vi "03_Perioda_frekvence_ze_spektra.vi"() -> ()   [LabVIEW 2019]
uses:
  <vilib>/Analysis/2dsp.llb/Real FFT.vi
  <vilib>/measure/NI_MABase.lvlib
  <vilib>/Analysis/NI_AALPro.lvlib
panel:
  out "Perioda signalu (s)":dbl=0.041666666666666664
  out "Frekvence signalu (Hz)":dbl=24.0
  out "SS (V)":dbl=2.573496971081113e-16
  in  "offset":dbl format="%0.2p"
  out "Spektrum":cluster{dbl[], dbl[]}(graph)
  out "Rozliseni a presnost spektra (Hz)":dbl=1.0
  out "Casovy prubeh":cluster{dbl[], dbl[]}(graph)
  out "dt (s)":dbl=0.0005
  out "Vzorkovaci Frekvence (N)":dbl=2000.0
  in  "Amplituda sumu":dbl format="%.2p"
  in  "Info o vzorkovani":T1={"Vzorkovaci frekvence"=2000.0, "Pocet vzorku v okne"=2000.0} {"Vzorkovaci frekvence" format="%.2p"}
  in  "Faze":dbl format="%.2p"
  in  "Amplituda":dbl=10.0 format="%0.2p"
  in  "Frekvence":dbl=24.0 format="%0.2p"
  # "GENEROVANI SIGNALU"
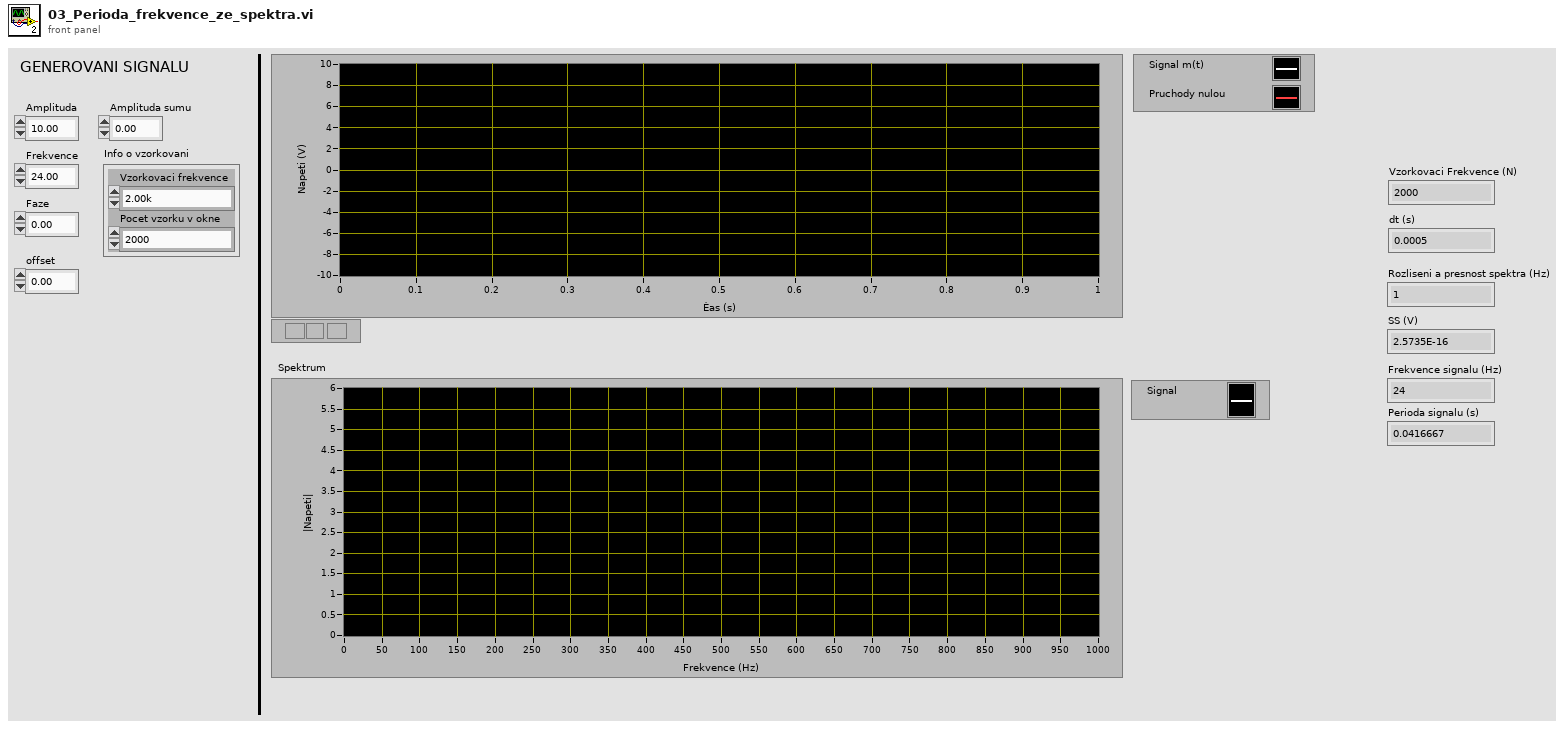
[diagram p1: front panel]
types:
  T1 = cluster{"Vzorkovaci frekvence":dbl, "Pocet vzorku v okne":dbl}
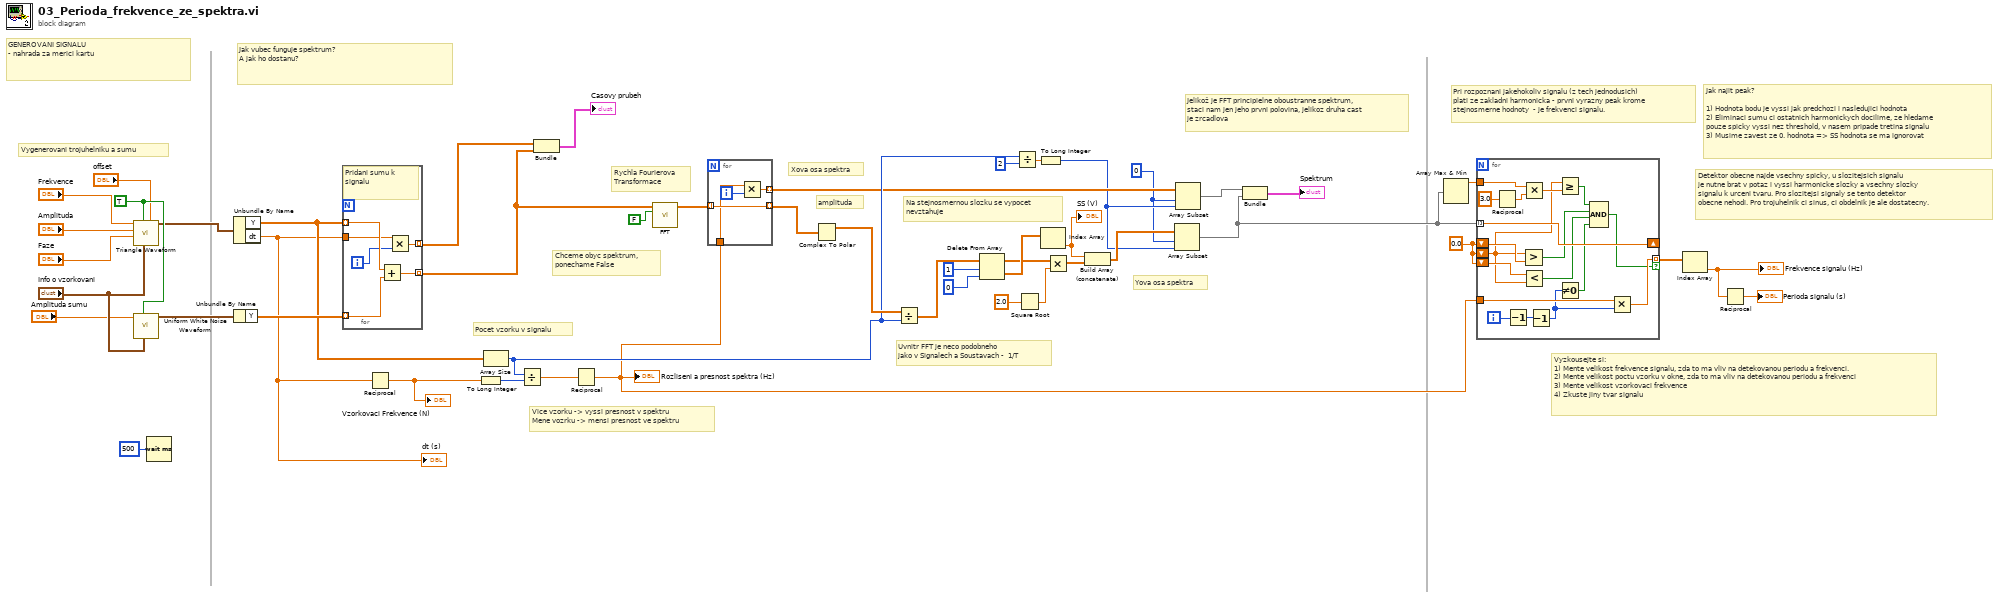
[diagram p0: block diagram]
diagram:
  w7 = 0.0
  w8 = 0 ("index")
  w43 = TRUE ("reset signal")
  # "Vyzkousejte si:\n1) Mente velikost frekvence signalu, zda to ma vliv na detekovanou periodu a frekvenci.\n2) Mente velikost poctu vzorku v okne, zda to ma vliv na detekovanou periodu a frekvenci\n3) Mente velikost vzorkovaci frekvence\n4) Zkuste jiny tvar signalu"
  # "Detektor obecne najde vsechny spicky, u slozitejsich signalu\nje nutne brat v potaz i vyssi harmonicke slozky a vsechny slozky\nsignalu k urceni tvaru. Pro slozitejsi signaly se tento detektor\nobecne nehodi. Pro trojuhelnik ci sinus, ci obdelnik je ale dostatecny."
  # "Jak najit peak?\n\n1) Hodnota bodu je vyssi jak predchozi i nasledujici hodnota\n2) Eliminaci sumu ci ostatnich harmonickych docilime, ze hledame\npouze spicky vyssi nez threshold, v nasem pripade tretina signalu\n3) Musime zavest ze 0. hodnota => SS hodnota se ma ignorovat"
  # "Pri rozpoznani jakehokoliv signalu (z tech jednodusich)\nplati ze zakladni harmonicka - prvni vyrazny peak krome \nstejnosmerne hodnoty  - je frekvenci signalu."
  # "Chceme obyc spektrum,\nponechame False"
  # "Vice vzorku -> vyssi presnost v spektru\nMene vozrku -> mensi presnost ve spektru"
  # "Jak vubec funguje spektrum?\nA jak ho dostanu?"
  # "Yova osa spektra"
  # "Xova osa spektra"
  # "Jelikož je FFT principielne oboustranne spektrum,\nstaci nam jen jeho prvni polovina, jelikoz druha cast\nje zrcadlova"
  # "Na stejnosmernou slozku se vypocet\nnevztahuje"
  # "Uvnitr FFT je neco podobneho\njako v Signalech a Soustavach -  1/T"
  # "amplituda"
  # "Rychla Fourierova\nTransformace"
  # "Pocet vzorku v signalu"
  # "GENEROVANI SIGNALU\n- nahrada za merici kartu"
  # "Vygenerovani trojuhelniku a sumu"
  n1 = call <vilib>:"Triangle Waveform.vi"("offset"="offset", "sampling info"="Info o vzorkovani", "reset signal"=w43, "phase"="Faze", "amplitude"="Amplituda", "frequency"="Frekvence") -> ("signal out"=w40:waveform(dbl))  [unwired: 4 in, 1 out]
  n2 = call <vilib>:"Uniform White Noise Waveform.vi"("sampling info"="Info o vzorkovani", "reset signal"=w43, "amplitude"="Amplituda sumu") -> ("signal out"=w42:waveform(dbl))  [unwired: 7 in, 1 out]
  n3 = Wait (ms)(milliseconds to wait=u32 500) -> ()  [unwired: 1 out]
  n4 = Unbundle By Name(w40) -> ("Y"=w36:dbl[], "dt"=w28:dbl)
  "dt (s)" <- w28
  n5 = Unbundle By Name(w42) -> ("Y"=w41:dbl[])
  n6 = for {
    tunnel: w36 -> [w53] mode=indexing
    tunnel: w41 -> [w54] mode=indexing
    tunnel: [w52] -> w27 mode=indexing
    tunnel: w28 -> [w51]
    tunnel: [w49] -> w38 mode=indexing
    i -> [w50]
    # "Pridani sumu k signalu"
    n7 = Add(x=w53, y=w54) -> (x+y=w52:dbl)
    n8 = Multiply(x=w51, y=w50) -> (x*y=w49:dbl)
  }
  n9 = Reciprocal(x=w28) -> (1/x=w35:dbl)
  "Vzorkovaci Frekvence (N)" <- w35
  n10 = To Long Integer(number=w35) -> (32bit integer=w34:i32)
  n11 = Array Size(array=w36) -> (size(s)=w17:i32)
  n12 = Divide(x=w17, y=w34) -> (x/y=w33:dbl)
  n13 = Bundle(w38, w27) -> (→"Casovy prubeh":cluster{dbl[], dbl[]})  [unwired: 1 in]
  n14 = Reciprocal(x=w33) -> (1/x=w6:dbl)
  "Rozliseni a presnost spektra (Hz)" <- w6
  n15 = call-poly <vilib>:"FFT.vi"("shift?"=FALSE, "X"=w27) -> ("FFT {X}"=w26:cdb[])  [unwired: 8 in, 1 out]
  n16 = for {
    tunnel: w26 -> [w57] mode=indexing
    tunnel: [w57] -> w32 mode=indexing
    tunnel: [w56] -> w14 mode=indexing
    tunnel: w6 -> [w55]
    i -> [w58]
    n17 = Multiply(x=w55, y=w58) -> (x*y=w56:dbl)
  }
  n18 = Complex To Polar(r * e^(i*theta)=w32) -> (r=w31:dbl[])  [unwired: 1 out]
  n19 = Divide(x=w31, y=w17) -> (x/y=w24:dbl[])
  n20 = Delete From Array(array=w24, length=1, index=0) -> (deleted portion=w21:dbl[], array with subset deleted=w20:dbl[])
  n21 = Divide(x=w17, y=2) -> (x/y=w15:dbl)
  n22 = Square Root(x=2.0) -> (sqrt(x)=w30:dbl)
  n23 = To Long Integer(number=w15) -> (32bit integer=w9:i32)
  n24 = Index Array(array=w21) -> (element=w19:dbl)  [unwired: 1 in]
  "SS (V)" <- w19
  n25 = Multiply(x=w20, y=w30) -> (x*y=w18:dbl[])
  n26 = Build Array (concatenate)(w19, w18) -> (w12:dbl[])
  n27 = Array Subset(array=w12, index=w8, length=w9) -> (w5:dbl[])
  n28 = Array Subset(array=w14, index=w8, length=w9) -> (w13:dbl[])
  n29 = Bundle(w13, w5) -> (→"Spektrum":cluster{dbl[], dbl[]})  [unwired: 1 in]
  n30 = Array Max & Min(array=w5) -> (max value=w4:dbl)  [unwired: 3 out]
  n31 = for {
    tunnel: w5 -> [w68] mode=indexing
    shift-right: [w68] -> _
    shift-left: w7 -> [w76]
    shift-left: w7 -> [w67]
    shift-left: w7 -> [w75]
    tunnel: [w73] -> w3 mode=indexing if=w61
    tunnel: w6 -> [w74]
    tunnel: w4 -> [w72]
    i -> [w66]
    n32 = Reciprocal(x=3.0) -> (1/x=w71:dbl)
    n33 = Decrement(x=w66) -> (x-1=w65:i32)
    n34 = Greater?(x=w67, y=w76) -> (0:w63:bool)
    n35 = Multiply(x=w72, y=w71) -> (x*y=w69:dbl)
    n36 = Less?(x=w75, y=w67) -> (x < y?=w62:bool)
    n37 = Decrement(x=w65) -> (x-1=w60:i32)
    n38 = Greater Or Equal?(x=w67, y=w69) -> (x >= y?=w64:bool)
    n39 = Not Equal To 0?(x=w60) -> (x != 0?=w59:bool)
    n40 = Compound Arithmetic op=AND(w64, w63, w62, w59) -> (w61:bool)
    n41 = Multiply(x=w74, y=w60) -> (x*y=w73:dbl)
  }
  n42 = Index Array(array=w3) -> (element=w2:dbl)  [unwired: 1 in]
  "Frekvence signalu (Hz)" <- w2
  n43 = Reciprocal(x=w2) -> (1/x=→"Perioda signalu (s)":dbl)
